vi "open calibration.vi"(6 "Folder":T1, 8 "error in (no error)":errorcluster, 11 "Index":u32) -> (0 "error out":errorcluster, 1 "file age":i32, 2 "conversion out":T12={"conversion matrix"=[[0.0, 0.0], [0.0, 0.0], [0.0, 0.0], [0.0, 0.0], [0.0, 0.0], [0.0, 0.0]], "units"="", "name"="", "scale type"=enum."Volts", "offset (volts)"=0.0, "second channel"=0, "correspondence table"=[], "offset (physical units)"=0.0, "pH scale"={"Buffers"=[], "Temperature"=0.0}, "D.O."={"Temperature"=0.0, "K"=0.0, "barometric pressure"=0.0}, "Photometer data"={"Dark Voltage"=0.0, "Blank Voltage"=0.0, "Standards"=[]}} {"D.O."."K" format="%.6f"; "D.O."."Temperature" format="%.2f"; "pH scale"."Buffers"."V/T" format="%.5f"; "pH scale"."Buffers"."Buffer" format="%.2f"; "pH scale"."Temperature" format="%.2f"; "offset (physical units)" format="%.5f"; "correspondence table"."volts" format="%.4f"; "correspondence table"."physical units" format="%.4f"; "second channel" min=-1; "offset (volts)" format="%.5f"; "conversion matrix" format="%.4e"})   [LabVIEW 2015]
uses:
  calibration/conversion.ctl
  DAQ configuration/scale type.ctl
  calibration/correspondence table.ctl
  calibration/pH/pH scale.ctl
  calibration/Dissolved Oxygen/DO scale.ctl
  calibration/Spectrophotometer/Photometer calibration data.ctl
  calibration/conversion 3.ctl
  Process Controller 3.0/Calibration and Function folders.ctl
  DAQ configuration/Sensor buffer command.ctl
panel:
  out "conversion out 2":T7={"conversion matrix"=[[0.0, 0.0], [0.0, 0.0], [0.0, 0.0], [0.0, 0.0], [0.0, 0.0], [0.0, 0.0]], "units"="", "name"="", "scale type"=enum."Volts", "offset (volts)"=0.0, "second channel"=0, "correspondence table"=[], "offset (physical units)"=0.0, "pH scale"={"Buffers"=[], "Temperature"=0.0}, "D.O."={"Temperature"=0.0, "K"=0.0, "barometric pressure"=0.0}, "Photometer data in"={"Dark Voltage"=0.0, "Blank Voltage"=0.0, "Standards"=[]}} {"D.O."."K" format="%.6f"; "D.O."."Temperature" format="%.2f"; "pH scale"."Buffers"."V/T" format="%.5f"; "pH scale"."Buffers"."Buffer" format="%.2f"; "pH scale"."Temperature" format="%.2f"; "offset (physical units)" format="%.5f"; "correspondence table"."volts" format="%.4f"; "correspondence table"."physical units" format="%.4f"; "second channel" min=-1; "offset (volts)" format="%.5f"; "conversion matrix" format="%.4e"}
  in  "Scale (prior to 11/12/15)":T8={"conversion matrix"=[[0.0, 0.0], [0.0, 0.0], [0.0, 0.0], [0.0, 0.0], [0.0, 0.0], [0.0, 0.0]], "units"="", "name"="", "scale type"=enum."Volts", "offset (volts)"=0.0, "second channel"=0, "correspondence table"=[], "offset (physical units)"=0.0, "pH scale"={"Buffers"=[], "Temperature"=0.0}, "D.O."={"Temperature"=0.0, "K"=0.0, "barometric pressure"=0.0}} {"D.O."."K" format="%.6f"; "D.O."."Temperature" format="%.2f"; "pH scale"."Buffers"."V/T" format="%.5f"; "pH scale"."Buffers"."Buffer" format="%.2f"; "pH scale"."Temperature" format="%.2f"; "offset (physical units)" format="%.5f"; "correspondence table"."volts" format="%.4f"; "correspondence table"."physical units" format="%.4f"; "second channel" min=-1; "offset (volts)" format="%.5f"; "conversion matrix" format="%.4e"}
  in  "conversion 3":T9={"conversion matrix"=[[0.0, 0.0], [0.0, 0.0], [0.0, 0.0], [0.0, 0.0], [0.0, 0.0], [0.0, 0.0]], "units"="", "name"="", "scale type"=enum."Volts", "offset (volts)"=0.0, "second channel"=0, "correspondence table"=[], "offset (physical units)"=0.0, "pH scale"={"Buffers"=[], "Temperature"=0.0}, "D.O."={"Temperature"=0.0, "K"=0.0}} {"D.O."."K" format="%.6f"; "D.O."."Temperature" format="%.2f"; "pH scale"."Buffers"."V/T" format="%.5f"; "pH scale"."Buffers"."Buffer" format="%.2f"; "pH scale"."Temperature" format="%.2f"; "offset (physical units)" format="%.5f"; "correspondence table"."volts" format="%.4f"; "correspondence table"."physical units" format="%.4f"; "second channel" min=-1; "offset (volts)" format="%.5f"; "conversion matrix" format="%.4e"}
  in  "conversion 2":T10={"conversion matrix"=[[0.0, 0.0], [0.0, 0.0], [0.0, 0.0], [0.0, 0.0], [0.0, 0.0], [0.0, 0.0]], "units"="", "name"="", "scale type"=enum."Volts", "offset (volts)"=0.0, "second channel"=0, "correspondence table"=[], "offset (physical units)"=0.0} {"offset (physical units)" format="%.5f"; "correspondence table"."volts" format="%.4f"; "correspondence table"."physical units" format="%.4f"; "second channel" min=-1; "offset (volts)" format="%.5f"; "conversion matrix" format="%.4e"}
  in  "conversion 1":T11={"conversion matrix"=[[0.0, 0.0], [0.0, 0.0], [0.0, 0.0], [0.0, 0.0], [0.0, 0.0], [0.0, 0.0]], "units"="", "name"="", "scale type"=enum."Volts", "offset (volts)"=0.0, "second channel"=0, "correspondence table"=[], "offset (physical units)"=0.0} {"offset (physical units)" format="%.5f"; "correspondence table"."volts" format="%.4f"; "correspondence table"."physical units" format="%.4f"; "second channel" min=-1; "offset (volts)" format="%.5f"; "conversion matrix" format="%.4e"}
  # "C"
  # "kPa"
  # "C"
  # "C"
  # "kPa"
  # "C"
  # "C"
  # "C"
  # "C"
  # "kPa"
  # "C"
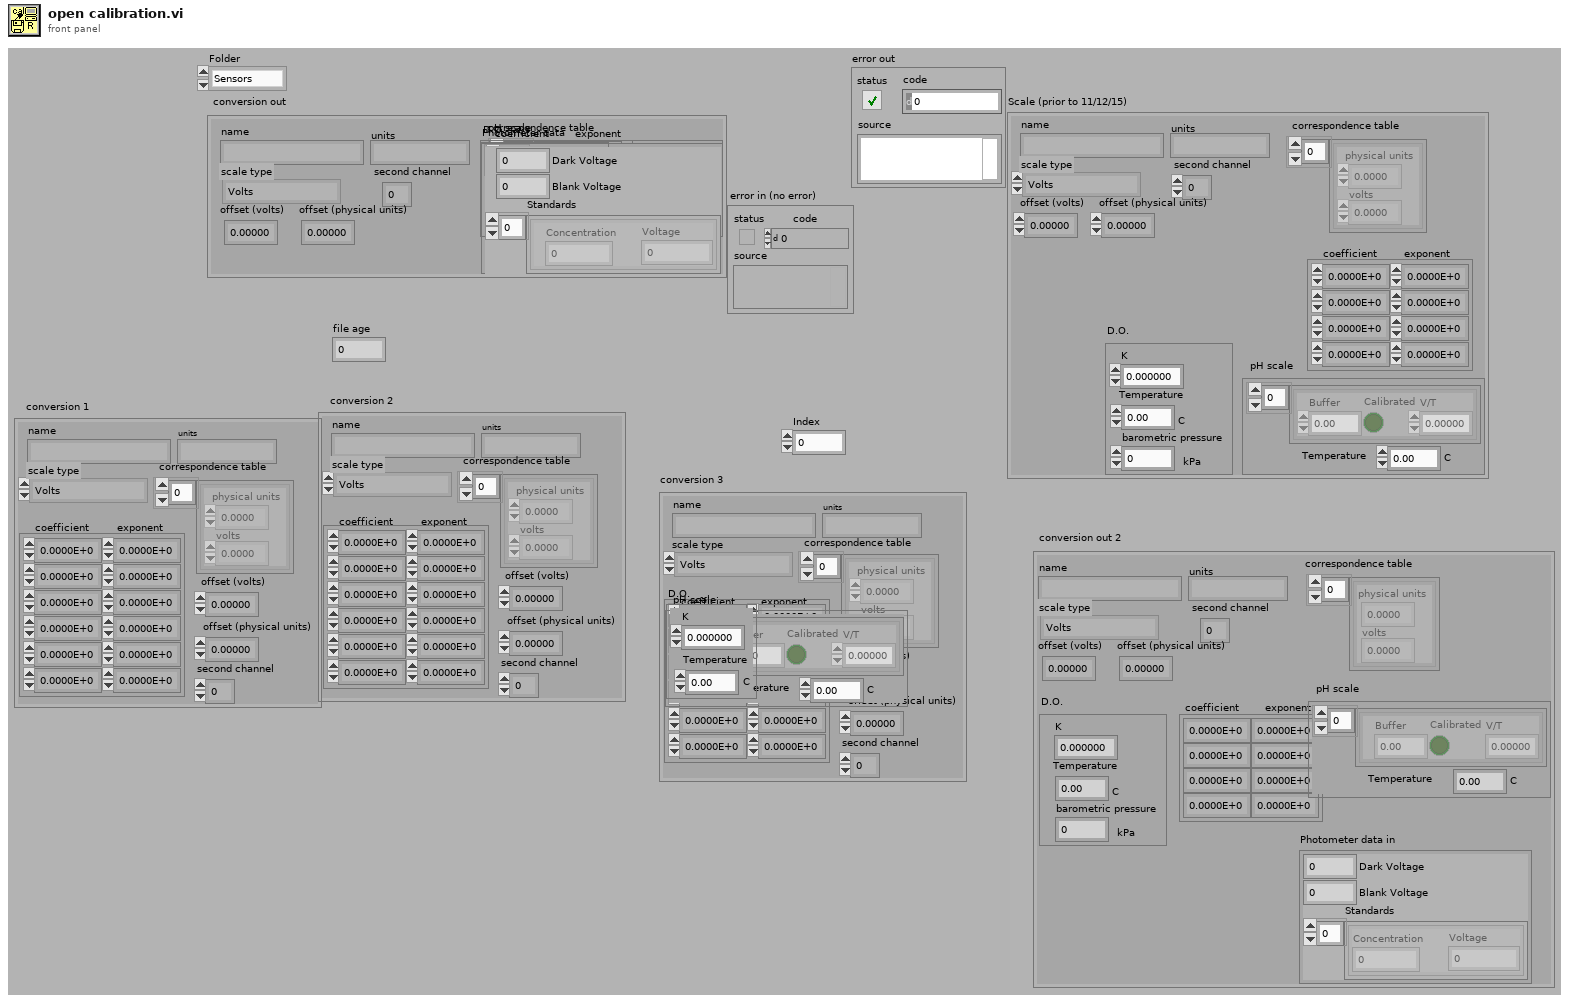
[diagram p1: front panel]
types:
  T1 = typedef "Calibration and Function folders.ctl" = enum16{"Sensors", "Functions", "Config File", "PublicAppFolder", "New ini File", "Set Config File", "Delete ini File"}
  T2 = typedef "scale type.ctl" = enum16{"Volts", "Polynomial", "Correspondence Table", "pH", "Dissolved Oxygen", "Quadratic", "Photometer"}
  T3 = typedef "correspondence table.ctl" = cluster{"physical units":dbl, "volts":dbl}[]
  T4 = typedef "pH scale.ctl" = cluster{"Buffers":cluster{"Buffer":dbl, "Calibrated":bool, "V/T":dbl}[], "Temperature":dbl}
  T5 = typedef "DO scale.ctl" = cluster{"Temperature":dbl, "K":dbl, "barometric pressure":dbl}
  T6 = typedef "Photometer calibration data.ctl" = cluster{"Dark Voltage":dbl, "Blank Voltage":dbl, "Standards":cluster{"Concentration":dbl, "Voltage":dbl}[]}
  T7 = cluster{"conversion matrix":sgl[][], "units":string, "name":string, "scale type":T2, "offset (volts)":dbl, "second channel":i8, "correspondence table":T3, "offset (physical units)":dbl, "pH scale":T4, "D.O.":T5, "Photometer data in":T6}
  T8 = cluster{"conversion matrix":sgl[][], "units":string, "name":string, "scale type":T2, "offset (volts)":dbl, "second channel":i8, "correspondence table":T3, "offset (physical units)":dbl, "pH scale":T4, "D.O.":T5}
  T9 = typedef "conversion 3.ctl" = cluster{"conversion matrix":sgl[][], "units":string, "name":string, "scale type":enum16{"Volts", "Polynomial", "Correspondence Table", "pH", "Dissolved Oxygen", "Quadratic"}, "offset (volts)":dbl, "second channel":i8, "correspondence table":cluster{"physical units":dbl, "volts":dbl}[], "offset (physical units)":dbl, "pH scale":cluster{"Buffers":cluster{"Buffer":dbl, "Calibrated":bool, "V/T":dbl}[], "Temperature":dbl}, "D.O.":cluster{"Temperature":dbl, "K":dbl}}
  T10 = cluster{"conversion matrix":sgl[][], "units":string, "name":string, "scale type":T2, "offset (volts)":dbl, "second channel":i8, "correspondence table":T3, "offset (physical units)":dbl}
  T11 = cluster{"conversion matrix":sgl[][], "units":string, "name":string, "scale type":enum16{"Volts", "Polynomial", "Correspondence Table", "pH", "Dissolved Oxygen"}, "offset (volts)":dbl, "second channel":i8, "correspondence table":T3, "offset (physical units)":dbl}
  T12 = typedef "conversion.ctl" = cluster{"conversion matrix":sgl[][], "units":string, "name":string, "scale type":T2, "offset (volts)":dbl, "second channel":i8, "correspondence table":T3, "offset (physical units)":dbl, "pH scale":T4, "D.O.":T5, "Photometer data":T6}
  T13 = typedef "Sensor buffer command.ctl" = enum16{"read average", "read recent", "read all", "write", "set buffer size", "Read channel config", "Write channel config", "clear"}
  T14 = enum16{"open", "open or create", "create or replace", "create", "open (read only)"}
  T15 = typedef "Channel config.ctl" = cluster{"Channel Indices":T16[], "AI Max voltage":dbl[], "Calibration matrix":T17}
  T16 = typedef "channel identifier.ctl" = u16
  T17 = typedef "calib array.ctl" = T12[]
  T18 = enum16{"read/write", "read-only", "write-only", "write-only (truncate)"}
  T19 = enum16{"Volts", "Polynomial", "Correspondence Table", "pH", "Dissolved Oxygen"}
  T20 = enum16{"Volts", "Polynomial", "Correspondence Table", "pH", "Dissolved Oxygen", "Quadratic"}
  T21 = cluster{"Buffers":cluster{"Buffer":dbl, "Calibrated":bool, "V/T":dbl}[], "Temperature":dbl}
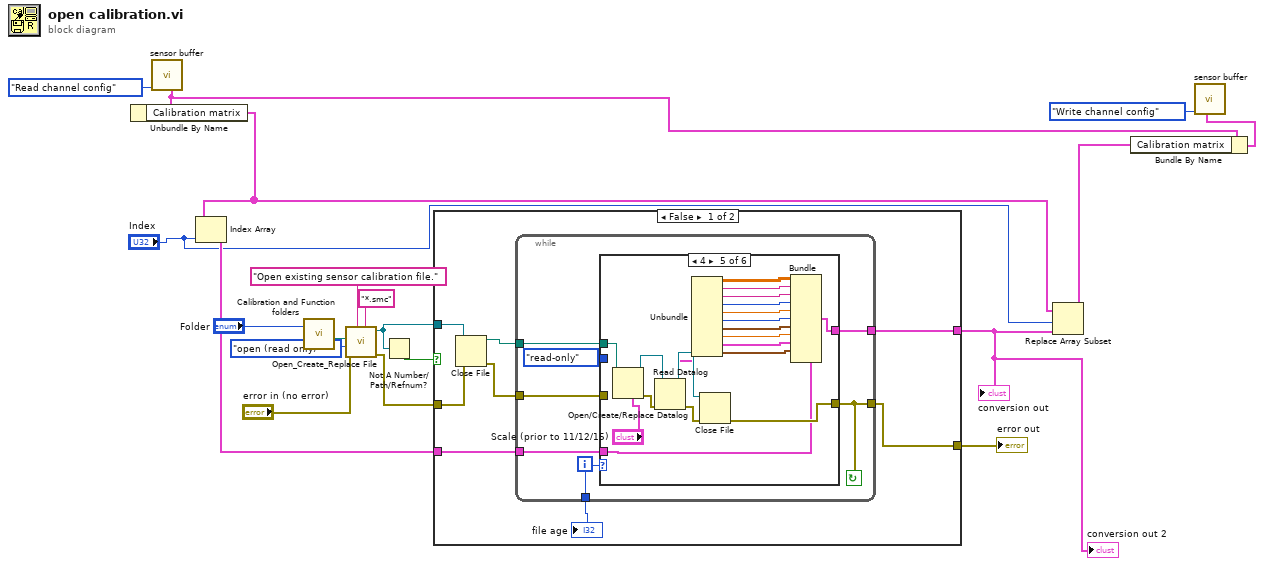
[diagram p0: block diagram]
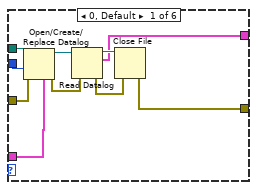
[diagram p2: hidden frame]
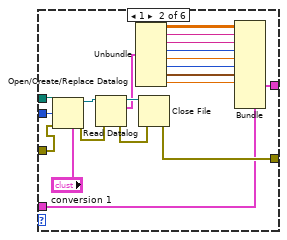
[diagram p3: hidden frame]
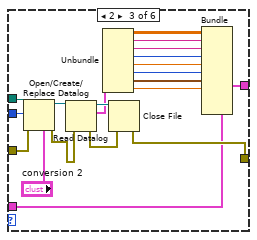
[diagram p4: hidden frame]
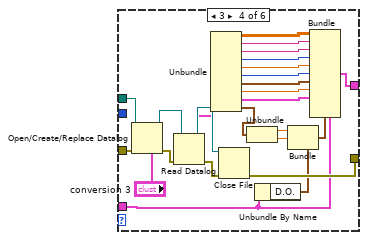
[diagram p5: hidden frame]
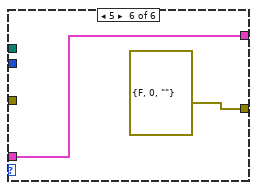
[diagram p6: hidden frame]
diagram:
  n1 = call "sensor buffer.vi"("command"=Sensor_buffer_command."Read channel config") -> ("Channel Config out"=w8:T15)  [unwired: 6 in, 4 out]
  n2 = Unbundle By Name(w8) -> ("Calibration matrix"=w10:T17)
  n3 = Index Array(array=w10, index="Index") -> (element=w13:T12)
  n4 = call "Calibration and Function folders.vi"("Folder"="Folder") -> ("Selected Folder"=w4:path)  [unwired: 9 in, 1 out]
  n5 = call <vilib>:"Open_Create_Replace File.vi"("pattern"="*.smc", "prompt"="Open existing sensor calibration file.", "error in (no error)"="error in (no error)", "function (open:0)"=T14."open (read only)", "start path  (Not A Path)"=w4) -> ("error out"=w15:errorcluster, "refnum"=w14:refnum<file>)  [unwired: 3 in, 2 out]
  n6 = Not A Number/Path/Refnum?(number/path/refnum=w14) -> (NaN/Path/Refnum?=w16:bool)
  n7 = case shown="False" w16 {
    tunnel: w14 -> [w27 _]
    tunnel: w15 -> [w26 w132]
    tunnel: [w24 w133] -> w5
    tunnel: w13 -> [w23 w133]
    tunnel: [w21 w132] -> w2
    frame False {
      n8 = Close File(refnum=w27, error in=w26) -> (path=w25:path, error out=w20:errorcluster)
      n9 = while {
        tunnel: [w34] -> w22
        tunnel: w23 -> [w29]
        tunnel: [w30] -> w24
        tunnel: [w31] -> w21
        tunnel: w25 -> [w32]
        tunnel: w20 -> [w28]
        i -> [w34]
        stop <- w31 continue-if-true
        n10 = case shown="4" w34 {
          tunnel: T18."read-only" ("open mode (0)") -> [w43 w63 w84 _ _ _]
          tunnel: w32 -> [w44 w64 w83 w98 w118 _]
          tunnel: [w38 w57 w77 w94 w114 errorcluster {"status"=FALSE, "code"=0, "source"=""} ("error out")] -> w31
          tunnel: [w37 w46 w74 w97 w117 w130] -> w30
          tunnel: w29 -> [w36 w47 w75 w87 w112 w130]
          tunnel: w28 -> [w35 w45 w65 w85 _ _]
          frame 0, Default {
            n11 = Open/Create/Replace Datalog(5:w36, 8:w35, 9:w43, 11:w44) -> (0:w39:errorcluster, 3:w40:refnum<k1>)  [unwired: 2 in, 1 out]
            n12 = Read Datalog(4:w39, 7:w40) -> (0:w41:errorcluster, 2:w37:T12, 3:w42:refnum<k1>)  [unwired: 1 in]
            n13 = Close File(refnum=w42, error in=w41) -> (error out=w38:errorcluster)  [unwired: 1 out]
          }
          frame 1 {
            n14 = Open/Create/Replace Datalog(5:"conversion 1", 8:w45, 9:w63, 11:w64) -> (0:w59:errorcluster, 3:w58:refnum<k1>)  [unwired: 2 in, 1 out]
            n15 = Read Datalog(4:w59, 7:w58) -> (0:w60:errorcluster, 2:w48:T11, 3:w61:refnum<k1>)  [unwired: 1 in]
            n16 = Unbundle(w48) -> ("conversion matrix"=w56:sgl[][], "units"=w55:string, "name"=w54:string, "scale type"=w53:T19, "offset (volts)"=w52:dbl, "second channel"=w51:i8, "correspondence table"=w50:T3, "offset (physical units)"=w49:dbl)
            n17 = Close File(refnum=w61, error in=w60) -> (error out=w57:errorcluster)  [unwired: 1 out]
            n18 = Bundle(cluster=w47, "conversion matrix"=w56, "units"=w55, "name"=w54, "scale type"=w53, "offset (volts)"=w52, "second channel"=w51, "correspondence table"=w50, "offset (physical units)"=w49) -> (w46:T12)  [unwired: 3 in]
          }
          frame 2 {
            n19 = Open/Create/Replace Datalog(5:"conversion 2", 8:w65, 9:w84, 11:w83) -> (0:w80:errorcluster, 3:w81:refnum<k1>)  [unwired: 2 in, 1 out]
            n20 = Read Datalog(4:w80, 7:w81) -> (0:w78:errorcluster, 2:w76:T10, 3:w79:refnum<k1>)  [unwired: 1 in]
            n21 = Unbundle(w76) -> ("conversion matrix"=w73:sgl[][], "units"=w72:string, "name"=w71:string, "scale type"=w70:T2, "offset (volts)"=w69:dbl, "second channel"=w68:i8, "correspondence table"=w67:T3, "offset (physical units)"=w66:dbl)
            n22 = Close File(refnum=w79, error in=w78) -> (error out=w77:errorcluster)  [unwired: 1 out]
            n23 = Bundle(cluster=w75, "conversion matrix"=w73, "units"=w72, "name"=w71, "scale type"=w70, "offset (volts)"=w69, "second channel"=w68, "correspondence table"=w67, "offset (physical units)"=w66) -> (w74:T12)  [unwired: 3 in]
          }
          frame 3 {
            n24 = Open/Create/Replace Datalog(5:"conversion 3", 8:w85, 11:w98) -> (0:w96:errorcluster, 3:w109:refnum<k1>)  [unwired: 3 in, 1 out]
            n25 = Read Datalog(4:w96, 7:w109) -> (0:w95:errorcluster, 2:w107:T9, 3:w108:refnum<k1>)  [unwired: 1 in]
            n26 = Unbundle(w107) -> ("conversion matrix"=w106:sgl[][], "units"=w105:string, "name"=w104:string, "scale type"=w103:T20, "offset (volts)"=w102:dbl, "second channel"=w101:i8, "correspondence table"=w100:cluster{"physical units":dbl, "volts":dbl}[], "offset (physical units)"=w99:dbl, "pH scale"=w93:T21, "D.O."=w91:cluster{"Temperature":dbl, "K":dbl})
            n27 = Close File(refnum=w108, error in=w95) -> (error out=w94:errorcluster)  [unwired: 1 out]
            n28 = Unbundle(w91) -> ("Temperature"=w89:dbl, "K"=w88:dbl)
            n29 = Unbundle By Name(w87) -> ("D.O."=w86:T5)
            n30 = Bundle(cluster=w86, "Temperature"=w89, "K"=w88) -> (w90:T5)  [unwired: 1 in]
            n31 = Bundle(cluster=w87, "conversion matrix"=w106, "units"=w105, "name"=w104, "scale type"=w103, "offset (volts)"=w102, "second channel"=w101, "correspondence table"=w100, "offset (physical units)"=w99, "pH scale"=w93, "D.O."=w90) -> (w97:T12)  [unwired: 1 in]
          }
          frame 4 {
            n32 = Open/Create/Replace Datalog(5:"Scale (prior to 11/12/15)", 11:w118) -> (0:w116:errorcluster, 3:w129:refnum<k1>)  [unwired: 4 in, 1 out]
            n33 = Read Datalog(4:w116, 7:w129) -> (0:w115:errorcluster, 2:w127:T8, 3:w128:refnum<k1>)  [unwired: 1 in]
            n34 = Unbundle(w127) -> ("conversion matrix"=w126:sgl[][], "units"=w125:string, "name"=w124:string, "scale type"=w123:T2, "offset (volts)"=w122:dbl, "second channel"=w121:i8, "correspondence table"=w120:T3, "offset (physical units)"=w119:dbl, "pH scale"=w113:T4, "D.O."=w110:T5)
            n35 = Close File(refnum=w128, error in=w115) -> (error out=w114:errorcluster)  [unwired: 1 out]
            n36 = Bundle(cluster=w112, "conversion matrix"=w126, "units"=w125, "name"=w124, "scale type"=w123, "offset (volts)"=w122, "second channel"=w121, "correspondence table"=w120, "offset (physical units)"=w119, "pH scale"=w113, "D.O."=w110) -> (w117:T12)  [unwired: 1 in]
          }
          frame 5 {
          }
        }
      }
      "file age" <- w22
    }
    frame True {
    }
  }
  "conversion out" <- w5
  "conversion out 2" <- w5
  "error out" <- w2
  n37 = Replace Array Subset(array=w10, new element=w5, index="Index") -> (w7:T17)
  n38 = Bundle By Name(cluster=w8, "Calibration matrix"=w7) -> (w6:T15)
  n39 = call "sensor buffer.vi"("Channel Config"=w6, "command"=Sensor_buffer_command."Write channel config") -> ()  [unwired: 5 in, 5 out]
